vi "TDT-Halt.vi"(0 "RPcoX":refnum<k7>, 11 "error in (no error)":errorcluster) -> (15 "error out":errorcluster)   [LabVIEW 2020]
doc: "Sets global variables that terminate the main DAQ loop."
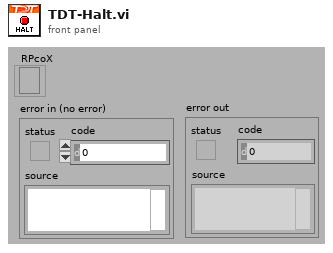
[diagram p1: front panel]
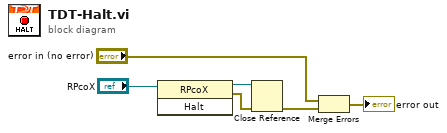
[diagram p0: block diagram]
diagram:
  n1 = invoke class="RPcoX" method="Halt"(reference="RPcoX") -> (reference out=w5:refnum<k7>, error out=w4:errorcluster)  [unwired: 2 in, 1 out]
  n2 = Close Reference(reference=w5, error in (no error)=w4) -> (error out=w3:errorcluster)
  n3 = Merge Errors("error in (no error)", w3) -> (→"error out":errorcluster)
